vi "Write_waveform.vi"(8 "error in (no error)":errorcluster, 9 "operation (0:open)":T1(ring)=enum."replace or create", 10 "Array":i8[](array[numeric]), 11 "Write_to_file in":refnum<class "Write_to_file.lvclass">) -> (0 "error out":errorcluster, 3 "Write_to_file out":refnum<class "Write_to_file.lvclass">)   [LabVIEW 2015, in "Write_to_file.lvclass"]
uses:
  Write_to_file.lvclass
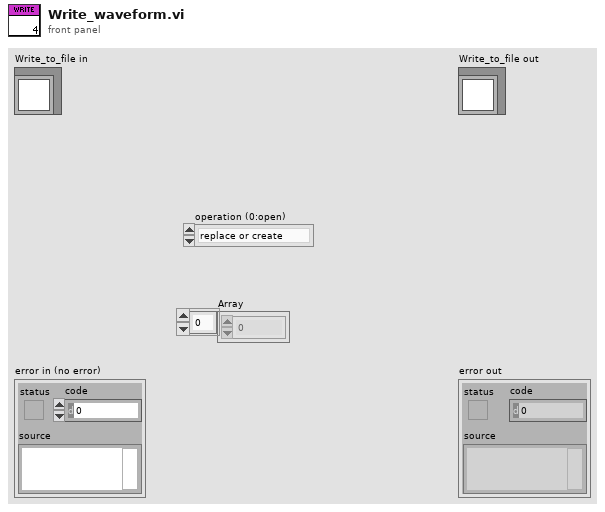
[diagram p1: front panel]
types:
  T1 = enum16{"open", "replace", "create", "open or create", "replace or create", "replace or create with confirmation"}
  T2 = enum16{"big-endian, network order", "native, host order", "little-endian"}
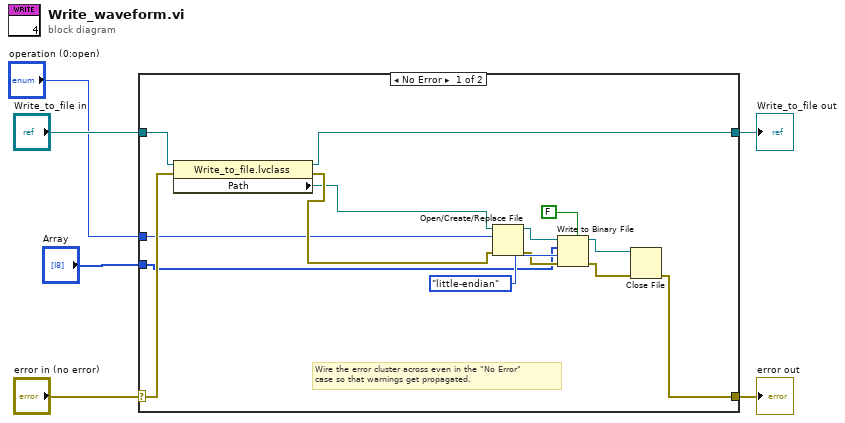
[diagram p0: block diagram]
diagram:
  n1 = case shown="No Error" "error in (no error)" {
    selector: "error in (no error)" -> [w18 w22]
    tunnel: [w10 w22] -> w5
    tunnel: [w19 w21] -> w3
    tunnel: "Write_to_file in" -> [w20 w21]
    tunnel: "Array" -> [w8 _]
    tunnel: "operation (0:open)" -> [w7 _]
    frame No Error {
      # "Wire the error cluster across even in the \"No Error\"\ncase so that warnings get propagated."
      n2 = property class="Write_to_file.lvclass"(reference=w20, error in=w18) -> (reference out=w19:refnum<class "Write_to_file.lvclass">, error out=w13:errorcluster, "Path"=w9:path)
      n3 = Open/Create/Replace File(file path (use dialog)=w9, error in=w13, operation (0:open)=w7) -> (refnum out=w17:refnum<file>, error out=w12:errorcluster)  [unwired: 3 in, 1 out]
      n4 = Write to Binary File(file (use dialog)=w17, data=w8, error in=w12, 5:FALSE ("prepend array or string size? (T)"), 9:T2."little-endian" ("byte order (0:big-endian, network order)")) -> (refnum out=w16:refnum<file>, error out=w11:errorcluster)  [unwired: 1 in, 1 out]
      n5 = Close File(refnum=w16, error in=w11) -> (error out=w10:errorcluster)  [unwired: 1 out]
    }
    frame Error {
    }
  }
  "error out" <- w5
  "Write_to_file out" <- w3
